vi "cipher users.vi"() -> (3 "password to cipher users":string)   [LabVIEW 2012]
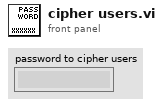
[diagram p1: front panel]
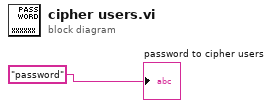
[diagram p0: block diagram]
diagram:
  "password to cipher users" <- "password" ("password to cipher users")
